vi "Add New XML Node.vi"(7 "Node Name":string, 8 "error in":errorcluster, 10 "Owning Element":refnum<k20>, 11 "DOM doc":refnum<k20>) -> (0 "error out":errorcluster, 2 "new element":refnum<k20>, 3 "DOM doc out":refnum<k20>)   [LabVIEW 2018, in "Serializer.lvclass"]
uses:
  Serializer.lvclass
  <resource>/objmgr/DOMUserDefRef.rc
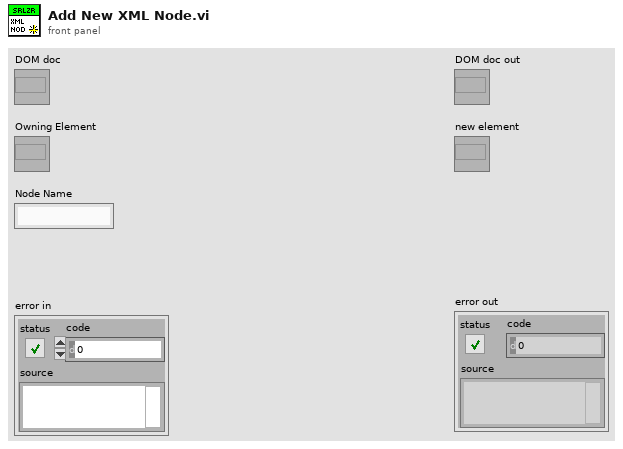
[diagram p1: front panel]
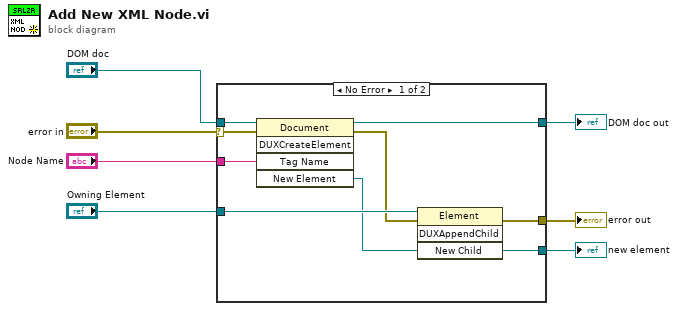
[diagram p0: block diagram]
diagram:
  n1 = case shown="No Error" "error in" {
    selector: "error in" -> [w12 w17]
    tunnel: "Node Name" -> [w15 _]
    tunnel: "DOM doc" -> [w14 w16]
    tunnel: "Owning Element" -> [w13 _]
    tunnel: [w11 w17] -> w5
    tunnel: [w8 _] -> w2
    tunnel: [w9 w16] -> w1
    frame No Error {
      n2 = invoke class="Document" method="DUXCreateElement"(reference=w14, error in=w12, "Tag Name"=w15) -> (reference out=w9:refnum<k20>, error out=w10:errorcluster, "New Element"=w8:refnum<k20>)  [unwired: 2 in, 2 out]
      n3 = invoke class="Element" method="DUXAppendChild"(reference=w13, error in=w10, "New Child"=w8) -> (error out=w11:errorcluster)  [unwired: 1 in, 3 out]
    }
    frame Error {
    }
  }
  "DOM doc out" <- w1
  "error out" <- w5
  "new element" <- w2
